vi "Frame_to_word_14444A.vi"() -> ()   [LabVIEW 2019]
uses:
  <vilib>/addons/Modulation/Analog/support/mod_Set Error Source.vi
  <vilib>/addons/Modulation/Digital/Support/Common/Validators/mod_Generate Filter Coefficients Validate.vi
  <vilib>/addons/Modulation/Digital/General/subVIs/mod_Generate Filter Coefficients.vi
  <vilib>/addons/Modulation/Digital/General/MT Generate ASK system parameters (M).vi
  <vilib>/addons/Modulation/Analog/MT Modulate AM (DSB).vi
  <vilib>/addons/Modulation/Analog/MT Upconvert Baseband (Real).vi
  <vilib>/measure/macond.llb/IIR Filter for 1 Chan.vi
  <vilib>/express/express analysis/Spectral/Block/exnSpectralBlock spectral measurements RMS poly.vi
  <vilib>/express/express analysis/Spectral/Block/exnSpectralBlock spectral measurements RMS WFM.vi
  <vilib>/addons/Modulation/Analog/MT Downconvert Passband (Real).vi
  <vilib>/addons/Modulation/Analog/MT Demodulate AM (DSB).vi
  <vilib>/ErrorRing/Error Ring.xnode
  <vilib>/express/express analysis/Spectral/XNode/ExpressSpectralMeasurementsBlockNode.xnode
  <vilib>/addons/Modulation/niAMT.lvlib
  <vilib>/measure/NI_MAPro.lvlib
  <vilib>/addons/Modulation/niDMT.lvlib
panel:
  out "error out":errorcluster
  out "Array of byte":u8[](array[numeric]) format="%x"
  out "SOF+DATA+EOF 3":cluster{"t0":dbl, "dt":dbl, "Y":dbl[]}(graph)
  out "Command":cluster{"t0":dbl, "dt":dbl, "Y":dbl[]}(graph)
  out "SOF+DATA+EOF 2":cluster{"t0":dbl, "dt":dbl, "Y":dbl[]}(graph)
  out "spectrum analog signal 6":waveform(dbl)(graph)
  out "spectrum analog signal 5":cluster{"t0":dbl, "dt":dbl, "Y":dbl[]}(graph)
  out "Analog signal 8":waveform(dbl)(graph)
  out "spectrum analog signal 4":cluster{"t0":dbl, "dt":dbl, "Y":dbl[]}(graph)
  out "Analog signal 9":waveform(dbl)(graph)
  out "Analog signal 7":waveform(dbl)(graph)
  out "Analog signal 4":waveform(dbl)(graph)
  in  "WUPA":u8[](array[numeric])=[82] format="%x"
  out "SOF+DATA+EOF":cluster{"t0":dbl, "dt":dbl, "Y":dbl[]}(graph)
  out "Video":cluster{"t0":dbl, "dt":dbl, "Y":dbl[]}(graph)
  out "video Miller":cluster{"t0":dbl, "dt":dbl, "Y":dbl[]}(graph)
  in  "command":enum16{"WUPA", "REQA"}(ring)
  out "spectrum analog signal 3":cluster{"t0":dbl, "dt":dbl, "Y":dbl[]}(graph)
  out "spectrum analog signal 2":cluster{"t0":dbl, "dt":dbl, "Y":dbl[]}(graph)
  out "spectrum analog signal":cluster{"t0":dbl, "dt":dbl, "Y":dbl[]}(graph)
  in  "CARRIER (hz)":dbl
  in  "BIT RATE":dbl
  out "100% ASK":waveform(dbl)(graph)
  in  "REQA":u8[](array[numeric])=[38] format="%x"
  # "REQA"
  # "WUPA"
  # "0"
  # "1"
  # "1"
  # "0"
  # "0"
  # "1"
  # "0"
  # "0"
  # "1"
  # "0"
  # "0"
  # "1"
  # "0"
  # "1"
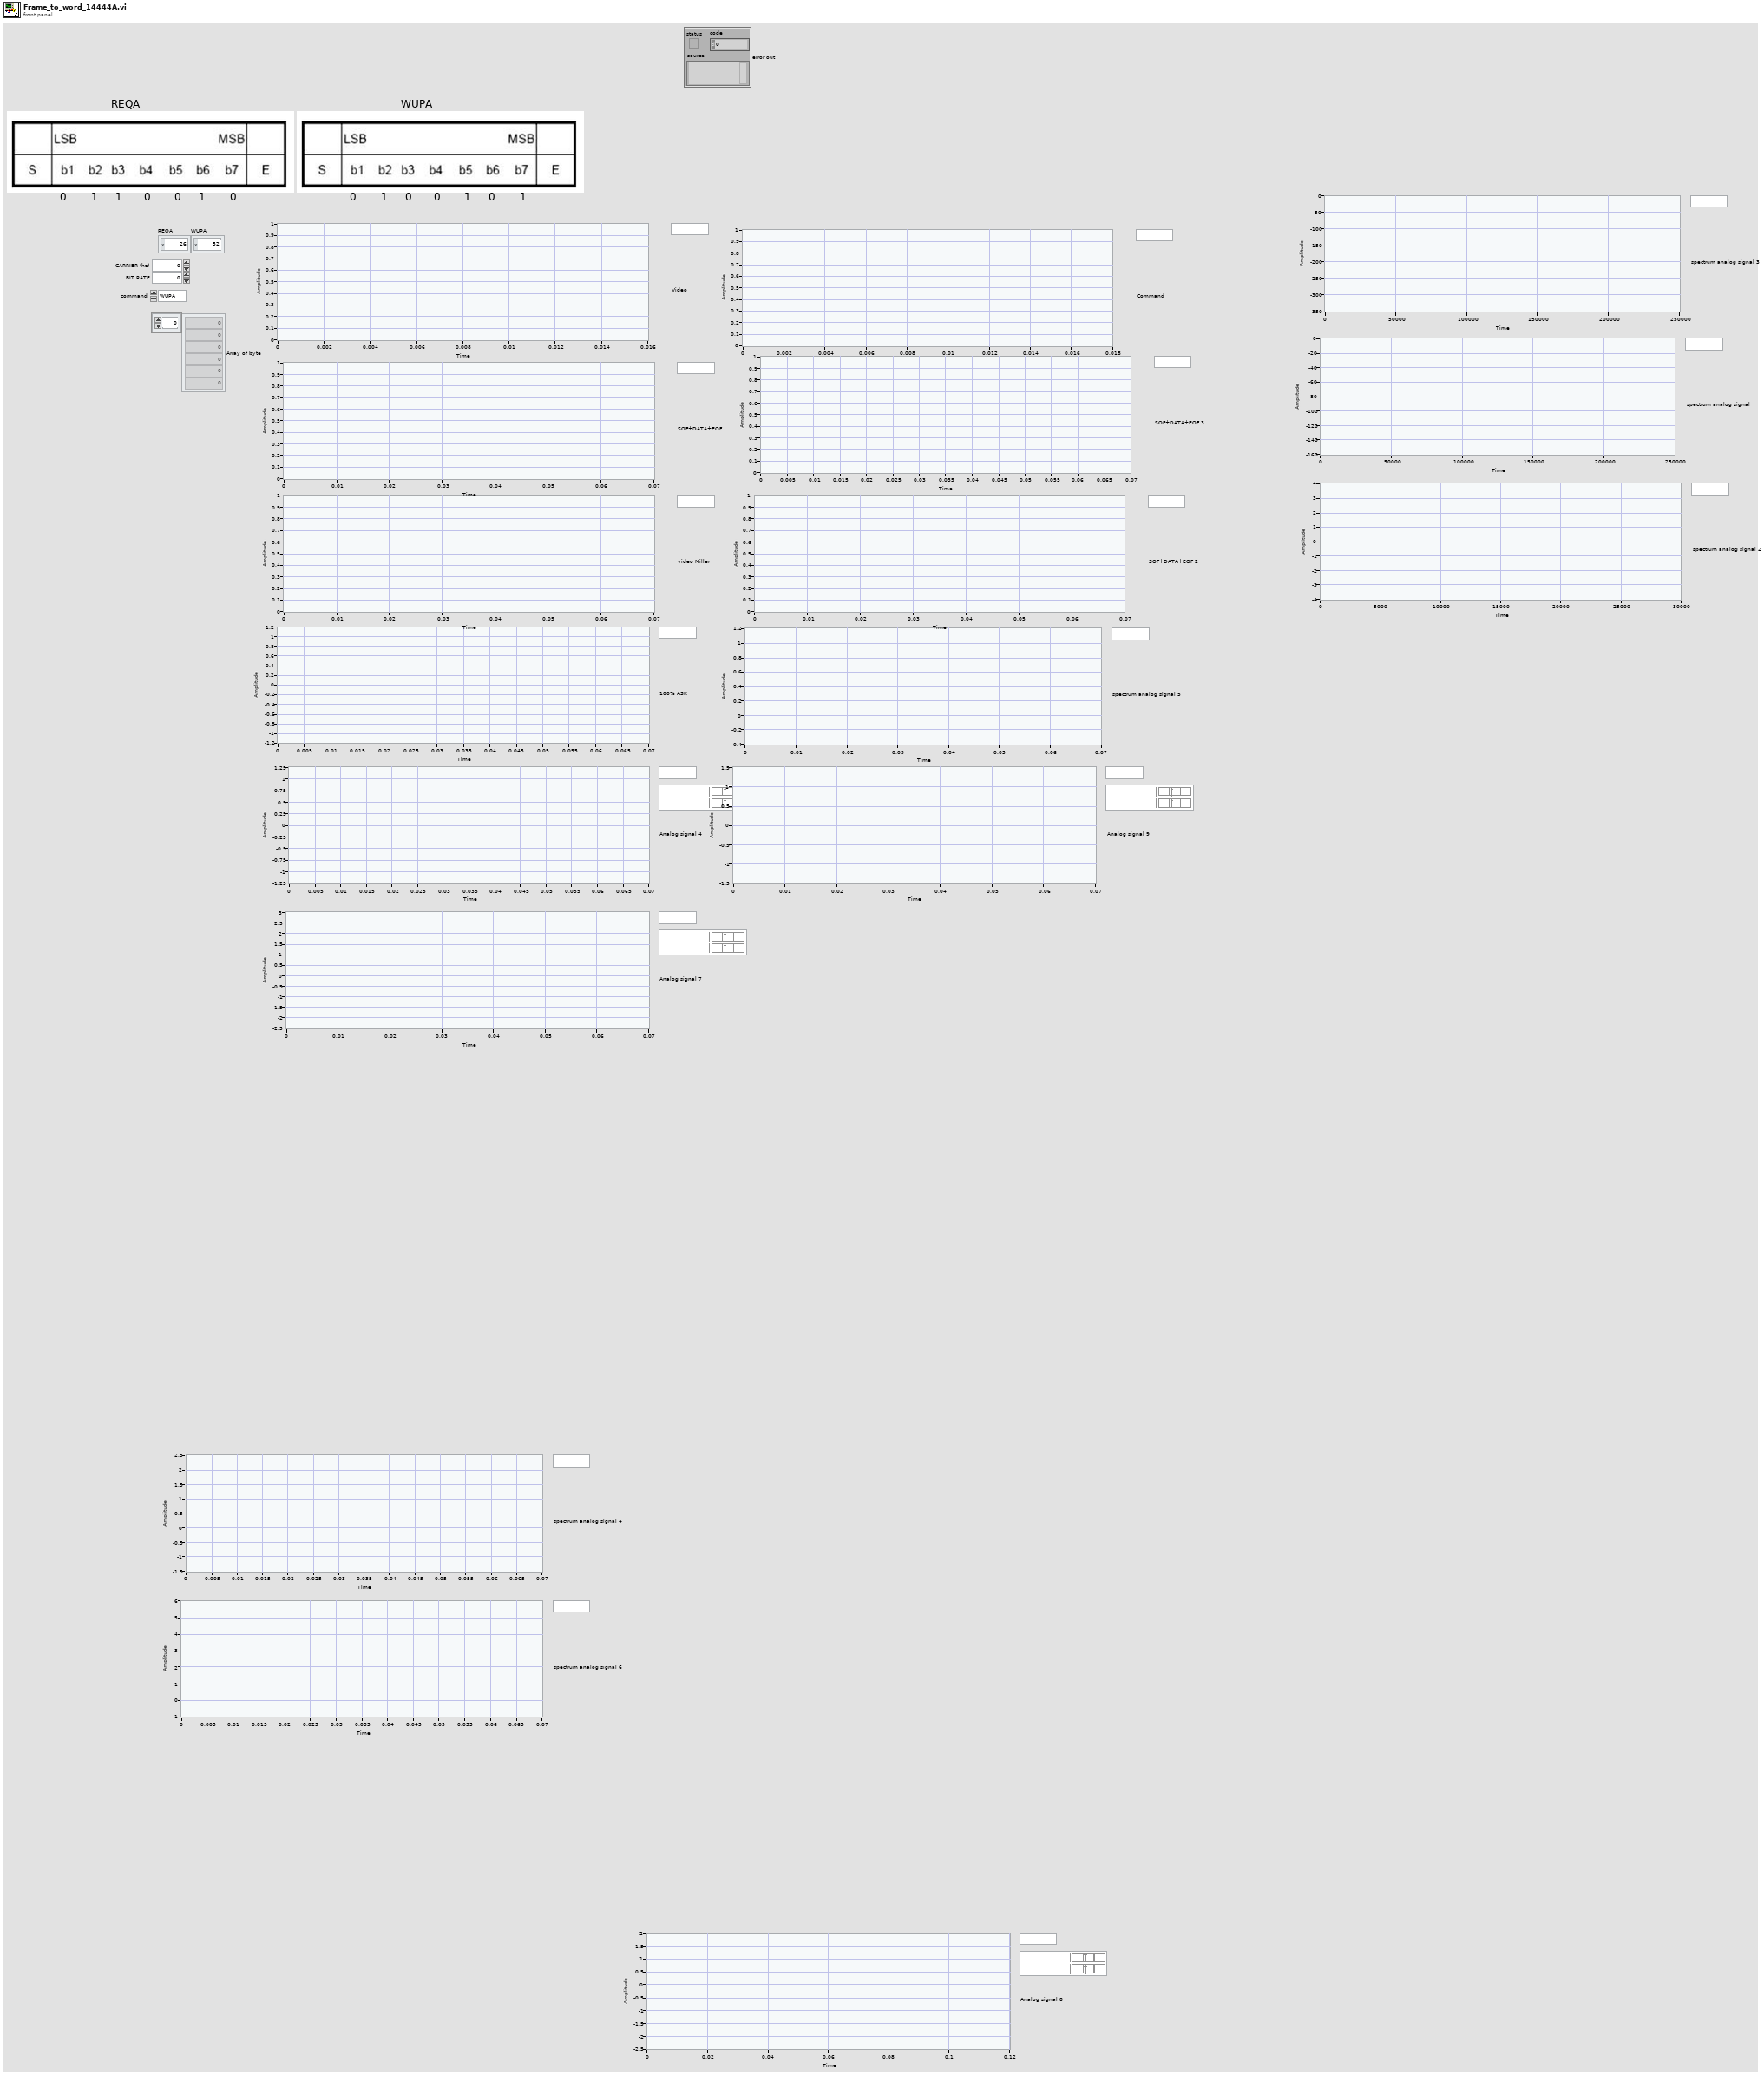
[diagram p1: front panel]
types:
  T1 = enum16{"none", "Raised Cosine", "Root Raised Cos", "Gaussian"}
  T2 = enum16{"FSK", "PSK", "QAM", "MSK", "PAM", "ASK", "CPM"}
  T3 = cluster{"passband ripple (dB)":dbl, "stopband start (Hz)":dbl, "stopband gain (dB)":dbl, "compute filter stopband ? (T)":bool}
  T4 = cluster{"Topology":enum16{"Off", "Butterworth", "Chebyshev", "Inverse Chebyshev", "Elliptic", "Bessel"}, "Type":enum16{"Lowpass", "Highpass", "Bandpass", "Bandstop"}, "Order":i32, "Lower Fc":dbl, "Upper Fc":dbl, "PB Ripple":dbl, "SB Attenuation":dbl}
  T5 = typedef "niAMT.lvlib/Complex Data Waveform.ctl" = cluster{"t0":dbl, "dt":dbl, "Y":cdb[]}
  T6 = cluster{"samples per symbol (16)":i32, "symbol map":cdb[]}
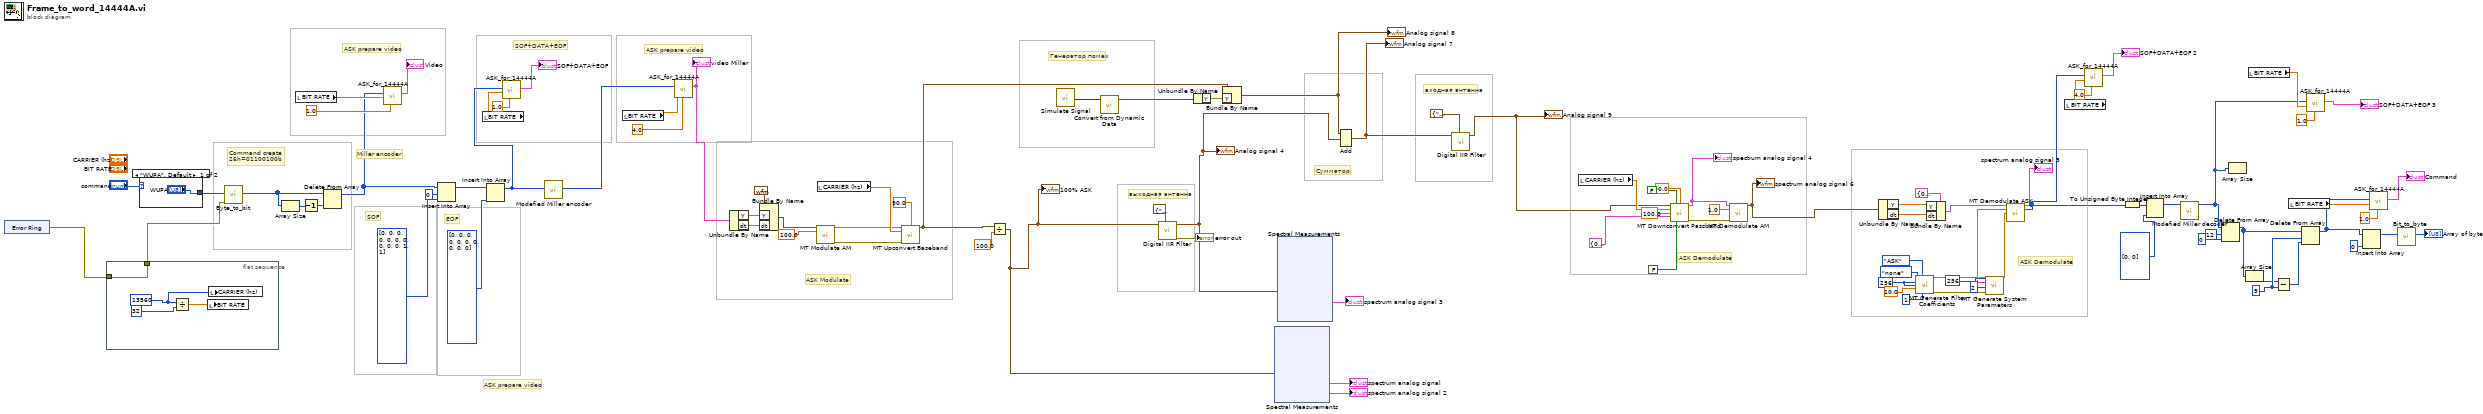
[diagram p0: block diagram]
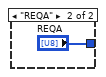
[diagram p2: hidden frame]
diagram:
  w20 = 9 ("length")
  w53 = 256 ("pulse shaping samples per symbol (16)")
  # "ASK prepare video"
  # "ASK Demodulate"
  # "ASK Demodulate"
  # "входная антенна"
  # "Сумматор"
  # "выходная антенна"
  # "Генератор помех"
  # "ASK Modulate"
  # "SOF+DATA+EOF"
  # "EOF"
  # "SOF"
  # "ASK prepare video"
  # "ASK prepare video"
  # "Miller encoder"
  # "Command create \n26h=01100100b"
  n1 = xnode "Error Ring"() -> ("error out"=w72:errorcluster)
  n2 = flat-sequence {
    tunnel: w72 -> [w98]
    tunnel: [w98] -> w71
    frame #0 {
      w99 = u32 13560
      n3 = Divide(x=w99, y=u32 32) -> (x/y=w100:dbl)
      n4 = local write "BIT RATE"(w100) -> ()
      n5 = local write "CARRIER (hz)"(w99) -> ()
    }
  }
  n6 = case shown="\"WUPA\", Default" "command" {
    tunnel: ["WUPA" "REQA"] -> w94
    frame "WUPA", Default {
    }
    frame "REQA" {
    }
  }
  n7 = call "Byte_to_bit.vi"("Error In"=w71, "Array of byte"=w94) -> ("Arrray of bit"=w97:u8[])  [unwired: 5 in, 2 out]
  n8 = Array Size(array=w97) -> (size(s)=w93:i32)
  n9 = local read "BIT RATE"() -> (w85:dbl)
  n10 = Decrement(x=w93) -> (x-1=w92:i32)
  n11 = Delete From Array(array=w97, index=w92) -> (array with subset deleted=w24:u8[])  [unwired: 1 in, 1 out]
  n12 = call "ASK_for_14444A.vi"("encoder divider"=1.0 ("y"), "BIT RATE"=w85, "Bit stream out (NRZ encode)"=w24) -> ("output complex waveform"=→"Video":T5)  [unwired: 7 in, 1 out]
  n13 = Insert Into Array(array=w24, index=0, new element=u8[] [0, 0, 0, 0, 0, 0, 0, 0, 0, 0, 1, 1] ("Bit stream out (NRZ encode)")) -> (w75:u8[])
  n14 = local read "BIT RATE"() -> (w80:dbl)
  n15 = Insert Into Array(array=w75, new element=u8[] [0, 0, 0, 0, 0, 0, 0, 0, 0, 0] ("Bit stream out (NRZ encode)")) -> (w16:u8[])  [unwired: 1 in]
  n16 = call "ASK_for_14444A.vi"("encoder divider"=1.0 ("y"), "BIT RATE"=w80, "Bit stream out (NRZ encode)"=w16) -> ("output complex waveform"=→"SOF+DATA+EOF":T5)  [unwired: 7 in, 1 out]
  n17 = call "Modefied Miller encoder.vi"("Bit stream in"=w16) -> ("Bit stream out (NRZ encode)"=w13:u8[])  [unwired: 9 in, 1 out]
  n18 = local read "BIT RATE"() -> (w96:dbl)
  n19 = call "ASK_for_14444A.vi"("encoder divider"=4.0 ("y"), "BIT RATE"=w96, "Bit stream out (NRZ encode)"=w13) -> ("output complex waveform"=w23:T5)  [unwired: 7 in, 1 out]
  "video Miller" <- w23
  n20 = Unbundle By Name(w23) -> ("Y"=w77:cdb[], "dt"=w76:dbl)
  n21 = Bundle By Name(cluster=waveform(cdb) {"t0"=timestamp(0 s since 1904-01-01), "dt"=1.0, "Y"=[]} ("waveform"), "Y"=w77, "dt"=w76) -> (w87:waveform(cdb))
  n22 = call-poly <vilib>:"MT Modulate AM.vi"("message signal"=w87, "modulation index"=100.0) -> ("AM modulated waveform"=w40:cluster{"t0":dbl, "dt":dbl, "Y":cdb[]}, "error out"=w89:errorcluster)  [unwired: 12 in]
  n23 = local read "CARRIER (hz)"() -> (w86:dbl)
  n24 = call-poly <vilib>:"MT Upconvert Baseband.vi"("baseband waveform (complex)"=w40, "initial phase (deg)"=90.0, "carrier frequency (Hz)"=w86, "error in (no error)"=w89) -> ("passband waveform"=w3:waveform(dbl))  [unwired: 10 in, 1 out]
  n25 = Divide(x=w3, y=100.0) -> (x/y=w2:waveform(dbl))
  "100% ASK" <- w2
  n26 = call "Simulate Signal"() -> ("Sine with Gaussian Noise"=w66:dynamicdata)  [unwired: 14 in, 1 out]
  n27 = call "Convert from Dynamic Data"("Dynamic Data Type"=w66) -> ("Waveform"=w65:waveform(dbl))  [unwired: 3 in]
  n28 = call-poly <vilib>:"Digital IIR Filter.vi"("IIR filter specifications"=T4 {"Topology"=enum."Butterworth", "Type"=enum."Bandpass", "Order"=3, "Lower Fc"=2000.0, "Upper Fc"=22000.0, "PB Ripple"=1.0, "SB Attenuation"=60.0}, "signal in"=w2) -> ("error out"=→"error out":errorcluster, "signal out"=w58:waveform(dbl))  [unwired: 7 in, 1 out]
  "Analog signal 4" <- w58
  n29 = Unbundle By Name(w65) -> ("Y"=w64:dbl[])
  n30 = Bundle By Name(cluster=w3, "Y"=w64) -> (w57:waveform(dbl))
  "Analog signal 8" <- w57
  n31 = xnode "Spectral Measurements"("Signals"=w2) -> ("FFT - (RMS)"=→"spectrum analog signal":cluster{"f0":dbl, "df":dbl, "magnitude":dbl[]}, "Phase"=→"spectrum analog signal 2":cluster{"f0":dbl, "df":dbl, "phase":dbl[]})  [unwired: 1 in, 1 out]
  n32 = xnode "Spectral Measurements"("Signals"=w58) -> ("FFT - (RMS)"=→"spectrum analog signal 3":cluster{"f0":dbl, "df":dbl, "magnitude":dbl[]})  [unwired: 1 in, 2 out]
  n33 = Add(1:w58, 2:w57) -> (0:w62:waveform(dbl))  [unwired: 1 in, 1 out]
  "Analog signal 7" <- w62
  n34 = call-poly <vilib>:"Digital IIR Filter.vi"("IIR filter specifications"=T4 {"Topology"=enum."Butterworth", "Type"=enum."Bandpass", "Order"=3, "Lower Fc"=2000.0, "Upper Fc"=22000.0, "PB Ripple"=1.0, "SB Attenuation"=60.0}, "signal in"=w62) -> ("signal out"=w39:waveform(dbl))  [unwired: 7 in, 2 out]
  "Analog signal 9" <- w39
  n35 = local read "CARRIER (hz)"() -> (w61:dbl)
  n36 = call-poly <vilib>:"MT Downconvert Passband.vi"("Waveform"=w39, "reset? (F)"=FALSE, "initial phase (deg)"=90.0, "carrier frequency (Hz)"=w61, "passband bandwidth (Hz)"=100.0, "advanced filter parameters"=T3 {"passband ripple (dB)"=0.01, "stopband start (Hz)"=0.0, "stopband gain (dB)"=-96.0, "compute filter stopband ? (T)"=TRUE}, "enable filter (T)"=FALSE) -> ("downconverted waveform (complex baseband)"=w35:T5, "error out"=w41:errorcluster)  [unwired: 5 in, 2 out]
  "spectrum analog signal 4" <- w35
  n37 = call-poly <vilib>:"MT Demodulate AM.vi"("AM modulated waveform"=w35, "modulation index"=1.0, "error in (no error)"=w41) -> ("AM demodulated waveform"=w4:waveform(dbl))  [unwired: 10 in, 2 out]
  "spectrum analog signal 6" <- w4
  n38 = Unbundle By Name(w4) -> ("Y"=w37:dbl[], "dt"=w36:dbl)
  n39 = call <vilib>:"MT Generate Filter Coefficients.vi"("pulse shaping filter (none)"=T1."none", "modulation type"=T2."ASK", "pulse shaping samples per symbol (16)"=w53, "matched samples per symbol (16)"=w53, "filter parameter"=10.0, "filter length (symbols)"=1) -> ("pulse shaping filter coefficients"=w47:dbl[], "error out"=w50:errorcluster)  [unwired: 1 in, 7 out]
  n40 = Bundle By Name(cluster=cluster{"t0":dbl, "dt":dbl, "Y":dbl[]} {"t0"=0.0, "dt"=0.0, "Y"=[]} ("AM modulated waveform"), "Y"=w37, "dt"=w36) -> (w34:cluster{"t0":dbl, "dt":dbl, "Y":dbl[]})
  n41 = call-poly <vilib>:"MT Generate System Parameters.vi"("samples per symbol (16)"=256, "M-ASK (2)"=2, "error in (no error)"=w50) -> ("ASK system parameters"=w48:T6)  [unwired: 12 out]
  n42 = call <vilib>:"MT Demodulate ASK.vi"("input complex waveform"=w34, "ASK system parameters"=w48, "matched filter coefficients"=w47) -> ("recovered complex waveform"=→"spectrum analog signal 5":T5, "output bit stream"=w28:i8[])  [unwired: 8 in, 3 out]
  n43 = local read "BIT RATE"() -> (w31:dbl)
  n44 = call "ASK_for_14444A.vi"("encoder divider"=4.0 ("y"), "BIT RATE"=w31, "Bit stream out (NRZ encode)"=w28) -> ("output complex waveform"=→"SOF+DATA+EOF 2":T5)  [unwired: 7 in, 1 out]
  n45 = To Unsigned Byte Integer(number=w28) -> (unsigned 8bit integer=w14:u8[])
  n46 = Insert Into Array(array=w14, new element=u8[] [0, 0]) -> (w12:u8[])  [unwired: 1 in]
  n47 = call "Modefied Miller decoder.vi"("Bit stream in"=w12) -> ("output array"=w15:u8[])  [unwired: 9 in, 1 out]
  n48 = Delete From Array(array=w15, length=12, index=0) -> (array with subset deleted=w22:u8[])  [unwired: 1 out]
  n49 = Array Size(array=w15) -> ()  [unwired: 1 out]
  n50 = Array Size(array=w22) -> (size(s)=w18:i32)
  n51 = local read "BIT RATE"() -> (w30:dbl)
  n52 = Subtract(x=w18, y=w20) -> (x-y=w19:i32)
  n53 = local read "BIT RATE"() -> (w25:dbl)
  n54 = Delete From Array(array=w22, length=w20, index=w19) -> (array with subset deleted=w9:u8[])  [unwired: 1 out]
  n55 = call "ASK_for_14444A.vi"("encoder divider"=1.0 ("y"), "BIT RATE"=w30, "Bit stream out (NRZ encode)"=w15) -> ("output complex waveform"=→"SOF+DATA+EOF 3":T5)  [unwired: 7 in, 1 out]
  n56 = Insert Into Array(array=w9, new element=u8 0 ("new element/subarray")) -> (w7:u8[])  [unwired: 1 in]
  n57 = call "ASK_for_14444A.vi"("encoder divider"=1.0 ("y"), "BIT RATE"=w25, "Bit stream out (NRZ encode)"=w9) -> ("output complex waveform"=→"Command":T5)  [unwired: 7 in, 1 out]
  n58 = call "Bit_to_byte.vi"("Array of bit"=w7) -> ("Array of byte"=→"Array of byte":u8[])  [unwired: 8 in, 2 out]
